vi "GateClose.vi"   [LabVIEW 2014, in "GateLib.lvlib"]
uses:
  GateLib.lvlib
  GateRefs.ctl
types:
  T1 = typedef "GateLib.lvlib/GateRefs.ctl" = enum16{"GateCyl"}
  T2 = typedef "WPI_SolenoidDevRef.ctl" = cluster{"DevStatus":errorcluster, "Pneumatics Control Module":u8, "Forward Solenoid Channel":T3, "Reverse Solenoid Channel":T3}
  T3 = typedef "WPI_SolenoidChannel.ctl" = enum8{"Solenoid 0", "Solenoid 1", "Solenoid 2", "Solenoid 3", "Solenoid 4", "Solenoid 5", "Solenoid 6", "Solenoid 7", "Invalid"}
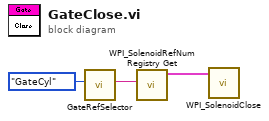
[diagram p0: block diagram]
diagram:
  n1 = call "GateRefSelector.vi"("GateRefs"=GateRefs."GateCyl") -> ("Refnum"=w3:string)  [unwired: 10 in]
  n2 = call <vilib>:"WPI_SolenoidRefNum Registry Get.vi"("refnum name"=w3) -> ("SolenoidDevRef"=w1:T2)  [unwired: 9 in, 1 out]
  n3 = call <vilib>:"WPI_SolenoidClose.vi"("SolenoidDevRef"=w1) -> ()  [unwired: 10 in, 1 out]
